vi "Enumerate.vi"(0 "object in":refnum<class "DFSTreeIterator.lvclass">, 5 "Error In":errorcluster) -> (14 "object out":refnum<class "DFSTreeIterator.lvclass">, 16 "Array":refnum<class "Node.lvclass">[](array[class]), 19 "Error Out":errorcluster)   [LabVIEW 2024, in "DFSTreeIterator.lvclass"]
uses:
  DFSTreeIterator.lvclass
  Node_class/Node.lvclass
  Support/Stack_class/Stack.lvclass
  DFSTreeIterator.lvclass/DFSTreeIterator.ctl
  Tree_class/Tree.lvclass
panel:
  # "Connector Pane"
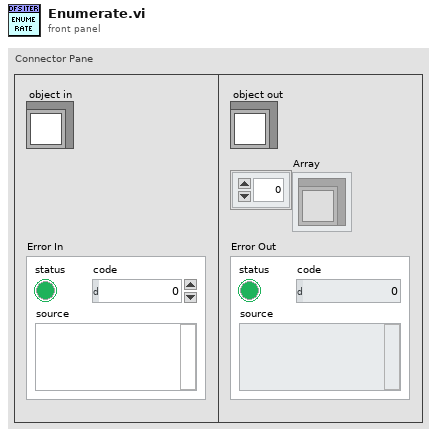
[diagram p1: front panel]
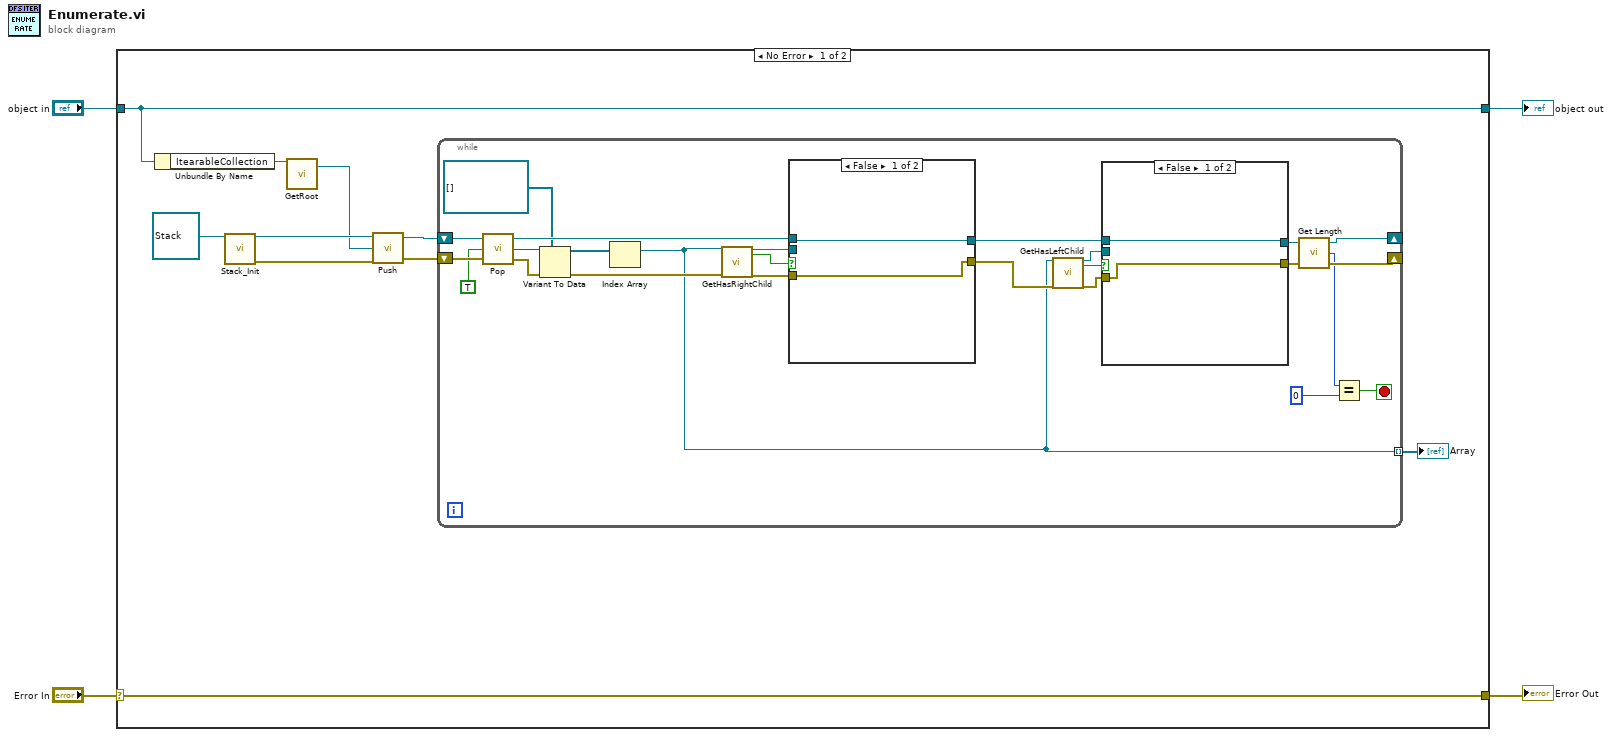
[diagram p0: block diagram]
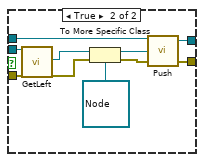
[diagram p2: hidden frame]
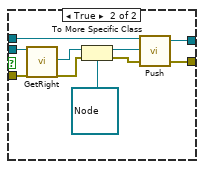
[diagram p3: hidden frame]
diagram:
  n1 = case shown="No Error" "Error In" {
    selector: "Error In" -> [w14 w65]
    tunnel: [w14 w65] -> w3
    tunnel: [w13 w64] -> w1
    tunnel: "object in" -> [w13 w64]
    frame No Error {
      n2 = Unbundle By Name(w13) -> ("ItearableCollection"=w9:refnum<class "Tree.lvclass">)
      n3 = call "Stack_Init.vi"("object in"=refnum<class "Stack.lvclass"> refnum ("Stack")) -> ("object out"=w10:refnum<class "Stack.lvclass">, "Error Out"=w11:errorcluster)  [unwired: 13 in]
      n4 = call-dynamic "GetRoot.vi"("object in"=w9) -> ("Root"=w8:refnum<class "Node.lvclass">)  [unwired: 16 in, 2 out]
      n5 = call-dynamic "Push.vi"("Error In"=w11, "Data"=w8, "object in"=w10) -> ("Error Out"=w6:errorcluster, "object out"=w7:refnum<class "Stack.lvclass">)  [unwired: 1 in]
      n6 = while {
        tunnel: [w15] -> w5 mode=indexing
        shift-right: [w22] -> _
        shift-left: w7 -> [w38]
        shift-right: [w24] -> _
        shift-left: w6 -> [w39]
        stop <- w21 stop-if-true
        n7 = call-dynamic "Pop.vi"("Error In"=w39, "Delete?"=TRUE, "object in"=w38) -> ("Error Out"=w35:errorcluster, "Data"=w36:variant, "object out"=w33:refnum<class "Stack.lvclass">)
        n8 = Variant To Data(error in=w35, type=refnum<class "Node.lvclass">[] [] ("Root"), Variant=w36) -> (data=w17:refnum<class "Node.lvclass">[], error out=w18:errorcluster)
        n9 = Index Array(array=w17) -> (element=w15:refnum<class "Node.lvclass">)  [unwired: 1 in]
        n10 = call-dynamic "GetHasRightChild.vi"("object in"=w15, "Error In"=w18) -> ("object out"=w32:refnum<class "Node.lvclass">, "HasRightChild"=w34:bool, "Error Out"=w31:errorcluster)  [unwired: 15 in]
        n11 = case shown="False" w34 {
          tunnel: w33 -> [w53 w63]
          tunnel: w32 -> [_ w55]
          tunnel: w31 -> [w52 w62]
          tunnel: [w52 w61] -> w28
          tunnel: [w53 w60] -> w29
          frame False {
          }
          frame True {
            n12 = call-dynamic "GetRight.vi"("object in"=w55, "Error In"=w62) -> ("Right"=w54:refnum<class "Element.lvclass">, "Error Out"=w56:errorcluster)  [unwired: 15 in, 1 out]
            n13 = To More Specific Class(target class=refnum<class "Node.lvclass"> refnum ("Node"), reference=w54, error in=w56) -> (specific class reference=w58:refnum<class "Node.lvclass">, error out=w59:errorcluster)
            n14 = call-dynamic "Push.vi"("Error In"=w59, "Data"=w58, "object in"=w63) -> ("Error Out"=w61:errorcluster, "object out"=w60:refnum<class "Stack.lvclass">)  [unwired: 1 in]
          }
        }
        n15 = call-dynamic "GetHasLeftChild.vi"("object in"=w15, "Error In"=w28) -> ("object out"=w26:refnum<class "Node.lvclass">, "HasLeftChild"=w27:bool, "Error Out"=w25:errorcluster)  [unwired: 15 in]
        n16 = case shown="False" w27 {
          tunnel: w29 -> [w41 w51]
          tunnel: w26 -> [_ w43]
          tunnel: w25 -> [w40 w50]
          tunnel: [w40 w49] -> w30
          tunnel: [w41 w48] -> w23
          frame False {
          }
          frame True {
            n17 = call-dynamic "GetLeft.vi"("object in"=w43, "Error In"=w50) -> ("Left"=w42:refnum<class "Element.lvclass">, "Error Out"=w44:errorcluster)  [unwired: 15 in, 1 out]
            n18 = To More Specific Class(target class=refnum<class "Node.lvclass"> refnum ("Node"), reference=w42, error in=w44) -> (specific class reference=w46:refnum<class "Node.lvclass">, error out=w47:errorcluster)
            n19 = call-dynamic "Push.vi"("Error In"=w47, "Data"=w46, "object in"=w51) -> ("Error Out"=w49:errorcluster, "object out"=w48:refnum<class "Stack.lvclass">)  [unwired: 1 in]
          }
        }
        n20 = call-dynamic "Get Length.vi"("Error In"=w30, "object in"=w23) -> ("Error Out"=w24:errorcluster, "Length"=w20:i32, "object out"=w22:refnum<class "Stack.lvclass">)  [unwired: 1 in]
        n21 = Equal?(x=w20, y=0) -> (x = y?=w21:bool)
      }
      "Array" <- w5
    }
    frame Error {
    }
  }
  "Error Out" <- w3
  "object out" <- w1
